vi "InitHelper.vi"(0 "object in":refnum<class "MTEC_Async.lvclass">, 5 "error in (no error)":errorcluster) -> (14 "object out":refnum<class "MTEC_Async.lvclass">, 19 "error out":errorcluster)   [LabVIEW 2019, in "MTEC_Async.lvclass"]
uses:
  MTEC_Async.lvclass
  MTEC_Async.lvclass/MTEC_Async.ctl
  TEC LabVIEW Control Software v0.14/Source/LV Source/Variables/FGVs/Type Defs/FGV_Operations.ctl
  TEC LabVIEW Control Software v0.14/Source/LV Source/[meerstetter engineering TE Cooling]/TypeDefs/meTEC_Configuration.ctl
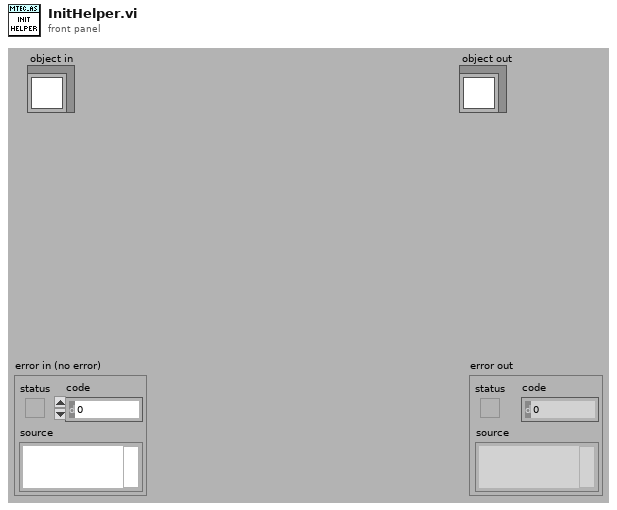
[diagram p1: front panel]
types:
  T1 = typedef "FGV_Operations.ctl" = enum16{"Read", "Write"}
  T2 = typedef "meTEC_Configuration.ctl" = cluster{"VISA resource name":refnum<visa-resource-name>, "Device Address":u16}
  T3 = typedef "FGV_TE Controller.ctl" = cluster{"SVs":cluster{"Unused":dbl}, "PVs":cluster{"FW & HW Versions":cluster{"Device Type [I32]":i32, "Device Type [String]":string, "Firmware Version [I32]":i32, "Firmware Version [String]":string, "Hardware Version [I32]":i32, "Hardware Version [String]":string, "Serial No.":i32}, "TEC Configuration":T2, "Object Target Temperature Source_CH1":u8, "Object Target Temperature Source_CH2":u8}, "Front Panel References":T4}
  T4 = typedef "FGV_Front Panel References.ctl" = cluster{"Main Loop Queue":refnum<queue>, "meTEC_Device Type":refnum<vi>, "meTEC_Serial No.":refnum<vi>, "meTEC_Hardware Version":refnum<vi>, "meTEC_Firmware Version":refnum<vi>, "meTEC_CH1_Object Target Temperature (ID 3000 / 50012) [°C]":refnum<vi>, "meTEC_CH1_Live Set Current (ID 50001) [A]":refnum<vi>, "meTEC_CH1_Live Set Voltage (ID 50002) [V]":refnum<vi>, "meTEC_CH1_Live Enable (ID 50000)":refnum<vi>, "meTEC_CH1_Input Selection (ID 2000)":refnum<vi>, "meTEC_CH1_Object Target Temp. Source Sel. (ID 50011)":refnum<vi>, "meTEC_CH2_Object Target Temperature (ID 3000 / 50012) [°C]":refnum<vi>, "meTEC_CH2_Live Set Current (ID 50001) [A]":refnum<vi>, "meTEC_CH2_Live Set Voltage (ID 50002) [V]":refnum<vi>, "meTEC_CH2_Live Enable (ID 50000)":refnum<vi>, "meTEC_CH2_Input Selection (ID 2000)":refnum<vi>, "meTEC_CH2_Object Target Temp. Source Sel. (ID 50011)":refnum<vi>, "meTEC_CH2_Object Temperature [°C]":refnum<vi>, "meTEC_CH2_Sink Temperature [°C]":refnum<vi>, "meTEC_CH2_Act. Output Current [A]":refnum<vi>, "meTEC_CH2_Act. Output Voltage [V]":refnum<vi>, "meTEC_CH2_Temperature Stability":refnum<vi>, "Monitor Chart_CH2":refnum<vi>, "meTEC_Initialize Device":refnum<vi>}
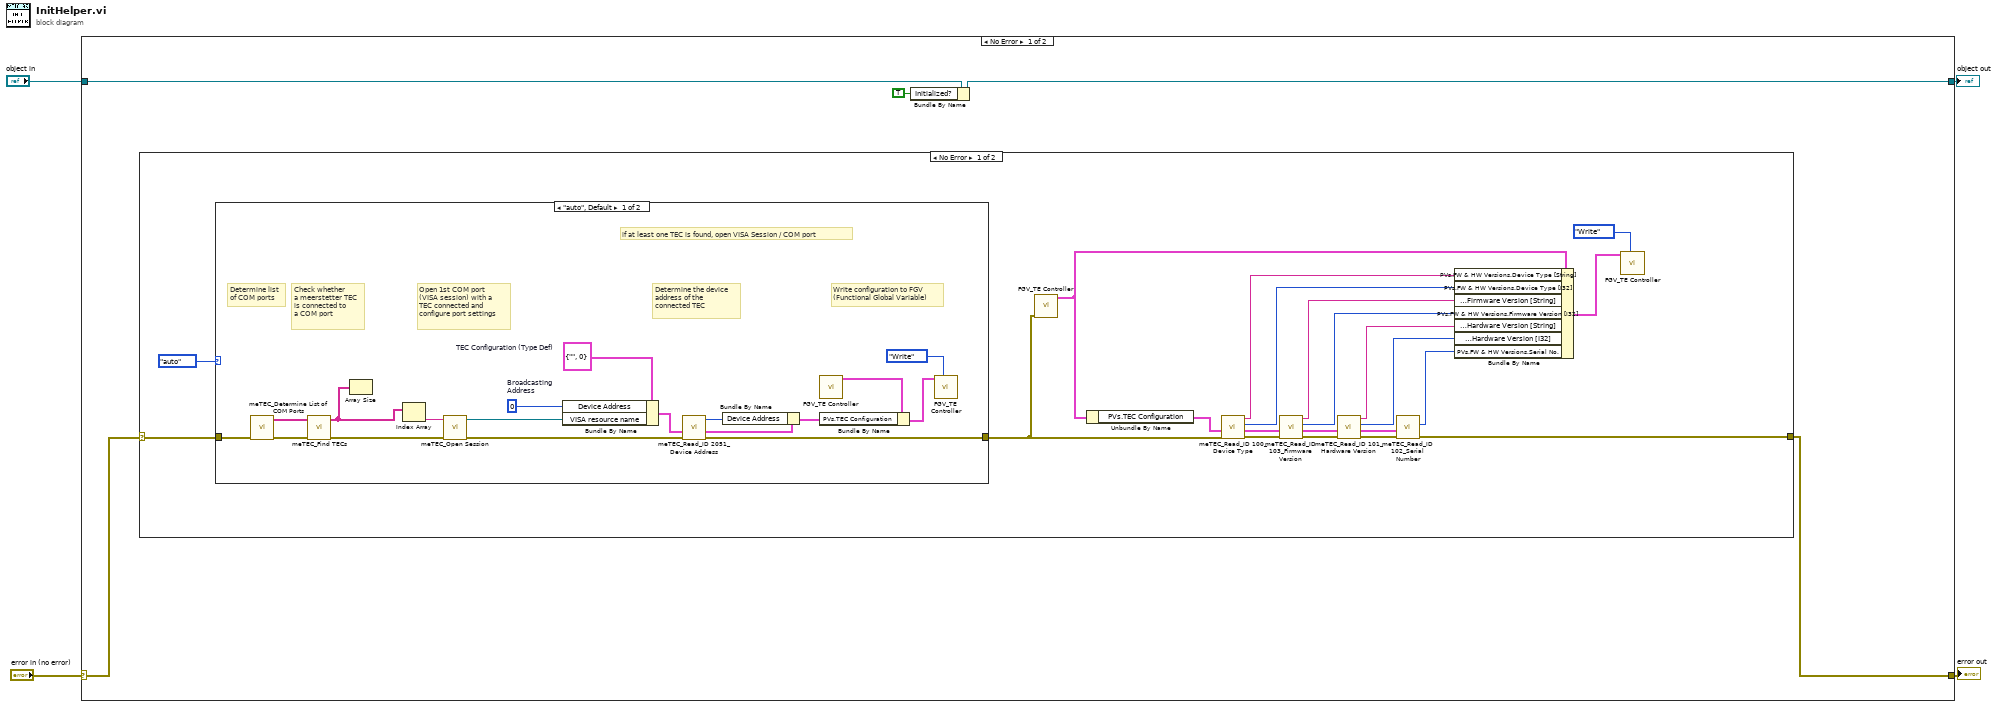
[diagram p0: block diagram]
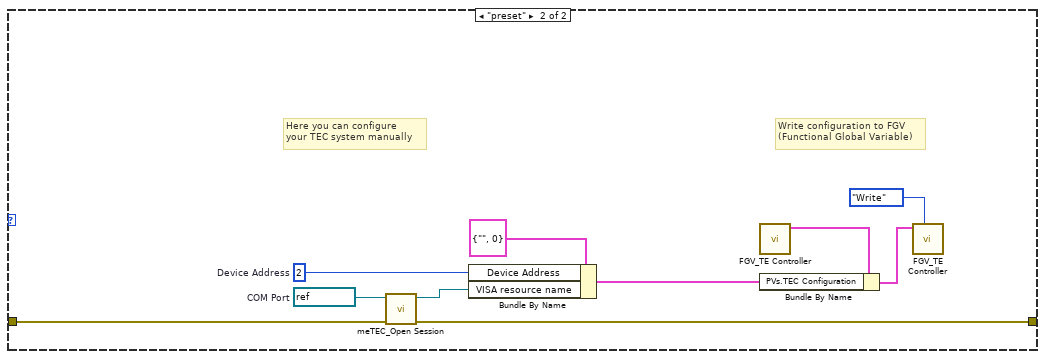
[diagram p2: hidden frame]
diagram:
  n1 = case shown="No Error" "error in (no error)" {
    selector: "error in (no error)" -> [w6 w61]
    tunnel: [w5 w61] -> w3
    tunnel: [w8 w60] -> w1
    tunnel: "object in" -> [w9 w60]
    frame No Error {
      n2 = case shown="No Error" w6 {
        selector: w6 -> [w12 w59]
        tunnel: [w10 w59] -> w5
        frame No Error {
          n3 = case shown="\"auto\", Default" enum16{"auto", "preset"}."auto" {
            tunnel: w12 -> [w45 w54]
            tunnel: [w31 w49] -> w11
            frame "auto", Default {
              w43 = T2 {"VISA resource name"="", "Device Address"=0}  # TEC Configuration (Type Def)
              w42 = u16 0  # Broadcasting  Address
              # "Write configuration to FGV\n(Functional Global Variable)"
              # "Determine the device\naddress of the \nconnected TEC"
              # "Open 1st COM port\n(VISA session) with a\nTEC connected and\nconfigure port settings"
              # "if at least one TEC is found, open VISA Session / COM port"
              # "Check whether\na meerstetter TEC\nis connected to\na COM port"
              # "Determine list\nof COM ports"
              n4 = call "meTEC_Determine List of COM Ports.vi"("error in (no error)"=w45) -> ("error out"=w48:errorcluster, "VISA Resources List (COM Ports)"=w47:string[])  [unwired: 9 in]
              n5 = call "meTEC_Find TECs.vi"("error in (no error)"=w48, "VISA Resources List (COM Ports)"=w47) -> ("error out"=w46:errorcluster, "VISA Resources List (meTEC(s))"=w44:string[])  [unwired: 8 in]
              n6 = Array Size(array=w44) -> ()  [unwired: 1 out]
              n7 = Index Array(array=w44) -> (element=w32:string)  [unwired: 1 in]
              n8 = call "meTEC_Open Session.vi"("error in (no error)"=w46, "COM Port"=w32) -> ("error out"=w41:errorcluster, "VISA resource name_OUT"=w40:refnum<visa-resource-name>)  [unwired: 8 in]
              n9 = Bundle By Name(cluster=w43, "Device Address"=w42, "VISA resource name"=w40) -> (w39:T2)
              n10 = call "meTEC_Read_ID 2051_Device Address.vi"("error in (no error)"=w41, "TEC Configuration_IN"=w39) -> ("error out"=w31:errorcluster, "TEC Configuration_OUT"=w37:T2, "Device Address (ID 2051) [I32]"=w38:i32)  [unwired: 7 in]
              n11 = Bundle By Name(cluster=w37, "Device Address"=w38) -> (w33:T2)
              n12 = call "FGV_TE Controller.vi"() -> ("FGV_TEC_OUT"=w36:T3)  [unwired: 10 in, 1 out]
              n13 = Bundle By Name(cluster=w36, "PVs.TEC Configuration"=w33) -> (w35:T3)
              n14 = call "FGV_TE Controller.vi"("Operation (Read)"=FGV_Operations."Write", "FGV_TEC_IN"=w35) -> ()  [unwired: 8 in, 2 out]
            }
            frame "preset" {
              w56 = u16 2  # Device Address
              w58 = refnum<visa-resource-name> "COM4"  # COM Port
              # "Here you can configure\nyour TEC system manually"
              # "Write configuration to FGV\n(Functional Global Variable)"
              n15 = call "meTEC_Open Session.vi"("error in (no error)"=w54, "COM Port"=w58) -> ("error out"=w49:errorcluster, "VISA resource name_OUT"=w55:refnum<visa-resource-name>)  [unwired: 8 in]
              n16 = Bundle By Name(cluster=T2 {"VISA resource name"="", "Device Address"=0} ("TEC Configuration"), "Device Address"=w56, "VISA resource name"=w55) -> (w50:T2)
              n17 = call "FGV_TE Controller.vi"() -> ("FGV_TEC_OUT"=w53:T3)  [unwired: 10 in, 1 out]
              n18 = Bundle By Name(cluster=w53, "PVs.TEC Configuration"=w50) -> (w52:T3)
              n19 = call "FGV_TE Controller.vi"("Operation (Read)"=FGV_Operations."Write", "FGV_TEC_IN"=w52) -> ()  [unwired: 8 in, 2 out]
            }
          }
          n20 = call "FGV_TE Controller.vi"("error in (no error)"=w11) -> ("FGV_TEC_OUT"=w25:T3)  [unwired: 9 in, 1 out]
          n21 = Unbundle By Name(w25) -> ("PVs.TEC Configuration"=w24:T2)
          n22 = call "meTEC_Read_ID 100_Device Type.vi"("error in (no error)"=w11, "TEC Configuration_IN"=w24) -> ("error out"=w28:errorcluster, "TEC Configuration_OUT"=w23:T2, "Device Type (ID 100) [I32]"=w14:i32, "Device Type (ID 100) [String]"=w15:string)  [unwired: 6 in]
          n23 = call "meTEC_Read_ID 103_Firmware Version.vi"("error in (no error)"=w28, "TEC Configuration_IN"=w23) -> ("error out"=w27:errorcluster, "TEC Configuration_OUT"=w22:T2, "Firmware Version (ID 103) [I32]"=w16:i32, "Firmware Version (ID 103) [String]"=w17:string)  [unwired: 6 in]
          n24 = call "meTEC_Read_ID 101_Hardware Version.vi"("error in (no error)"=w27, "TEC Configuration_IN"=w22) -> ("error out"=w26:errorcluster, "TEC Configuration_OUT"=w21:T2, "Hardware Version (ID 101) [I32]"=w18:i32, "Hardware Version (ID 101) [String]"=w19:string)  [unwired: 6 in]
          n25 = call "meTEC_Read_ID 102_Serial Number.vi"("error in (no error)"=w26, "TEC Configuration_IN"=w21) -> ("error out"=w10:errorcluster, "Serial No. (ID 102) [I32]"=w20:i32)  [unwired: 6 in, 2 out]
          n26 = Bundle By Name(cluster=w25, "PVs.FW & HW Versions.Device Type [String]"=w15, "PVs.FW & HW Versions.Device Type [I32]"=w14, "PVs.FW & HW Versions.Firmware Version [String]"=w17, "PVs.FW & HW Versions.Firmware Version [I32]"=w16, "PVs.FW & HW Versions.Hardware Version [String]"=w19, "PVs.FW & HW Versions.Hardware Version [I32]"=w18, "PVs.FW & HW Versions.Serial No."=w20) -> (w30:T3)
          n27 = call "FGV_TE Controller.vi"("Operation (Read)"=FGV_Operations."Write", "FGV_TEC_IN"=w30) -> ()  [unwired: 8 in, 2 out]
        }
        frame Error {
        }
      }
      n28 = Bundle By Name(cluster=w9, "Initialized?"=TRUE) -> (w8:refnum<class "MTEC_Async.lvclass">)
    }
    frame Error {
    }
  }
  "error out" <- w3
  "object out" <- w1
